vi "GetCurrentPosition.vi"() -> ()   [LabVIEW 2009]
uses:
  <vilib>/Instr/_visa.llb/VISA Configure Serial Port (Instr).vi
panel:
  out "In Range?":bool
  in  "COM PORT":refnum<visa-resource-name>
  out "Current Values":u32
  out "number":u32
  out "substring":string
  out "VISA resource name out 2":refnum<visa-resource-name>
  out "error out 2":errorcluster
  out "read buffer":string
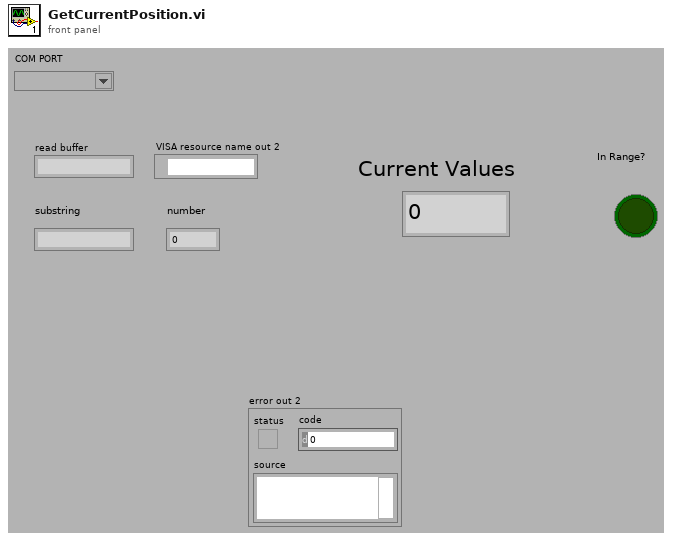
[diagram p1: front panel]
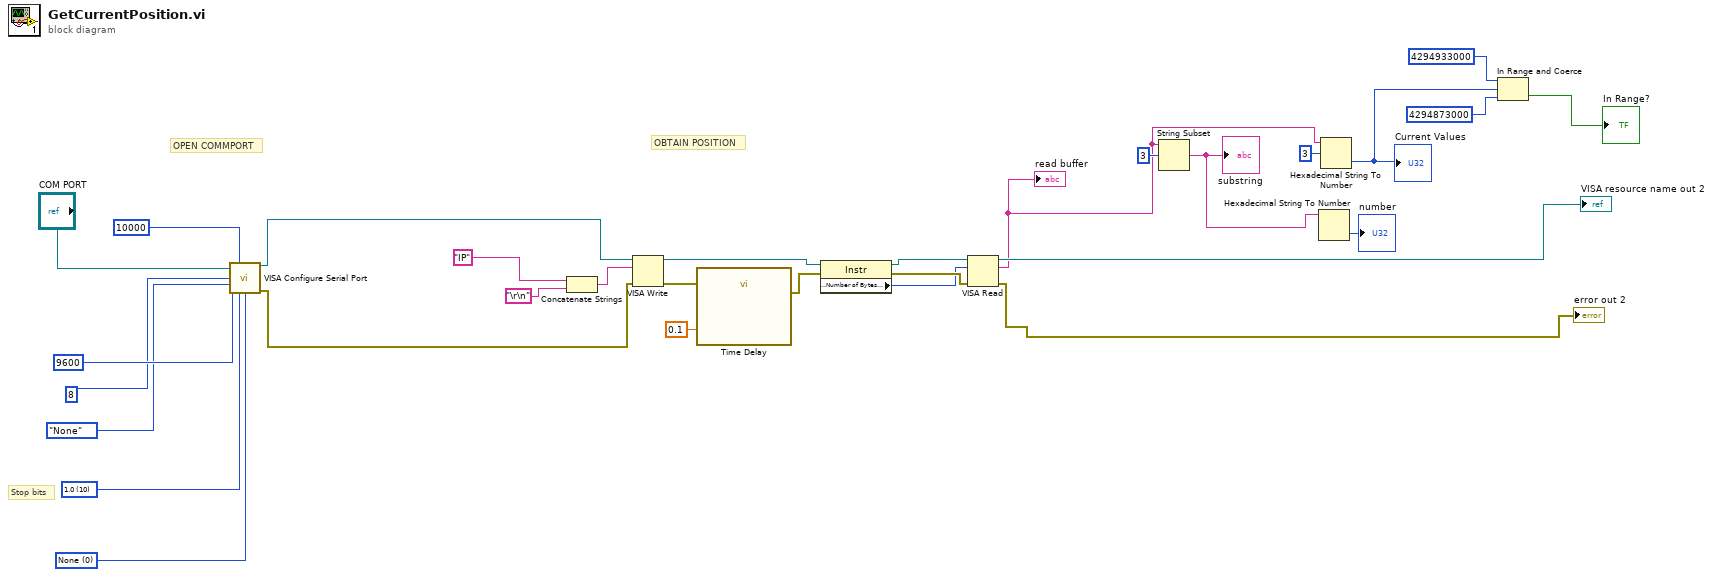
[diagram p0: block diagram]
diagram:
  w8 = u16 0 items=["None", "XON/XOFF", "RTS/CTS", "XON/XOFF & RTS/CTS", "DTR/DSR", "XON/XOFF & DTR/DSR"] ("flow control (0:none)")
  w9 = u16 10 items=["1.0"=10, "1.5"=15, "2.0"=20] ("stop bits (10: 1 bit)")
  # "OBTAIN POSITION"
  # "Stop bits"
  # "OPEN COMMPORT"
  n1 = call-poly "VISA Configure Serial Port"("VISA resource name"="COM PORT", "timeout (10sec)"=u32 10000, "baud rate (9600)"=u32 9600, "data bits (8)"=u16 8, "parity (0:none)"=enum16{"None", "Odd", "Even", "Mark", "Space"}."None", "stop bits (10: 1 bit)"=w9, "flow control (0:none)"=w8) -> ("VISA resource name out"=w7:refnum<visa-resource-name>, "error out"=w6:errorcluster)  [unwired: 7 in]
  n2 = Concatenate Strings("IP" ("string"), "\r\n") -> (w26:string)
  n3 = VISA Write(VISA resource name=w7, write buffer=w26, error in (no error)=w6) -> (VISA resource name out=w30:refnum<visa-resource-name>, error out=w24:errorcluster)  [unwired: 1 out]
  n4 = call "Time Delay"("error in (no error)"=w24, "Delay Time (s)"=0.1) -> ("error out"=w23:errorcluster)  [unwired: 9 in]
  n5 = property class="Instr"(reference=w30, error in=w23) -> (reference out=w28:refnum<visa-resource-name>, error out=w29:errorcluster, "Serial Settings:Number of Bytes at Serial Port"=w27:u32)
  n6 = VISA Read(VISA resource name=w28, byte count=w27, error in (no error)=w29) -> (VISA resource name out=→"VISA resource name out 2":refnum<visa-resource-name>, read buffer=w14:string, error out=→"error out 2":errorcluster)  [unwired: 1 out]
  "read buffer" <- w14
  n7 = String Subset(string=w14, offset (0)=3) -> (substring=w15:string)  [unwired: 1 in]
  "substring" <- w15
  n8 = Hexadecimal String To Number(string=w15) -> (number=→"number":u32)  [unwired: 2 in, 1 out]
  n9 = Hexadecimal String To Number(string=w14, offset=3) -> (number=w4:u32)  [unwired: 1 in, 1 out]
  "Current Values" <- w4
  n10 = In Range and Coerce(upper limit=u32 4294933000, x=w4, lower limit=u32 4294873000) -> (In Range?=→"In Range?":bool)  [unwired: 1 out]
